vi "RFFE Extended Register Write Example.vi"() -> ()   [LabVIEW 2018]
uses:
  Slave Address.ctl
  Register Address.ctl
  Register Data.ctl
  MIPI RFFE API.lvlib
panel:
  in  "Register Data":T1[](array[typedef]) format="%02x"
  in  "Register Address":T2 format="%02x"
  in  "Slave Address":T3=12 format="%02x"
  in  "Bus Number":i32
  in  "Resource Name":refnum<k15>
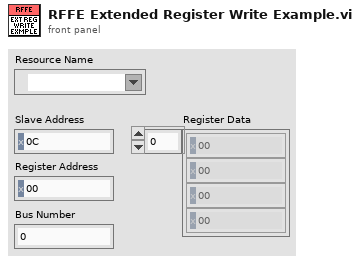
[diagram p1: front panel]
types:
  T1 = typedef "MIPI RFFE API.lvlib/Register Data.ctl" = u8
  T2 = typedef "MIPI RFFE API.lvlib/Register Address.ctl" = u16
  T3 = typedef "MIPI RFFE API.lvlib/Slave Address.ctl" = u8
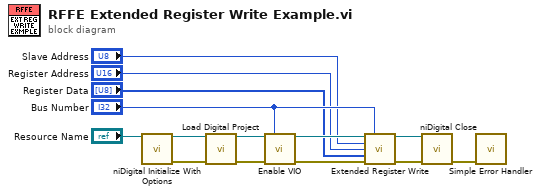
[diagram p0: block diagram]
diagram:
  n1 = call <instrlib>:"niDigital Initialize With Options.vi"("resource name"="Resource Name") -> ("instrument handle"=w6:refnum<k15>, "error out"=w5:errorcluster)  [unwired: 13 in]
  n2 = call "Load Digital Project.vi"("instrument handle"=w6, "error in"=w5) -> ("instrument handle out"=w14:refnum<k15>, "error out"=w13:errorcluster)  [unwired: 12 in]
  n3 = call "Enable VIO.vi"("instrument handle"=w14, "Bus Number"="Bus Number", "error in"=w13) -> ("instrument handle out"=w10:refnum<k15>, "error out"=w8:errorcluster)  [unwired: 11 in]
  n4 = call "Extended Register Write.vi"("instrument handle in"=w10, "Bus Number"="Bus Number", "Slave Address"="Slave Address", "Register Address"="Register Address", "Register Data"="Register Data", "error in (no error)"=w8) -> ("instrument handle out"=w9:refnum<k15>, "error out"=w7:errorcluster)  [unwired: 8 in]
  n5 = call <instrlib>:"niDigital Close.vi"("instrument handle"=w9, "error in"=w7) -> ("error out"=w11:errorcluster)  [unwired: 13 in]
  n6 = call <vilib>:"Simple Error Handler.vi"("error in (no error)"=w11) -> ()  [unwired: 4 in, 5 out]
